vi "GetErrorStructureSize.vi"(8 "error in (no error)":errorcluster) -> (0 "error out":errorcluster, 3 "CS size if BD is empty":T1={"Width (%)"=70.0, "Height (%)"=50.0})   [LabVIEW 2017, in "ErrorStructureDrawer.lvlib"]
doc: "Gets the size at which the new case structure should be drawn if there is nothing to put inside that case structure from the config FGV. Size is specified as a percentage of the size of the visible block diagram."
uses:
  ErrorStructureDrawer.lvlib
  Controls/CaseStructureSizeIfBD_Empty.ctl
  Controls/GetSetCommand.ctl
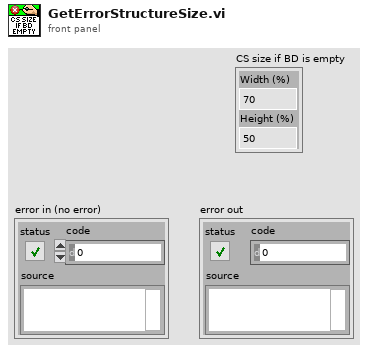
[diagram p1: front panel]
types:
  T1 = typedef "ErrorStructureDrawer.lvlib/CaseStructureSizeIfBD_Empty.ctl" = cluster{"Width (%)":dbl, "Height (%)":dbl}
  T2 = typedef "ErrorStructureDrawer.lvlib/GetSetCommand.ctl" = enum16{"Get", "Set"}
  T3 = typedef "ErrorStructureDrawer.lvlib/ErrorStructureDrawerSettings.ctl" = cluster{"Error control config":T4, "BD alignment settings":T5, "Case structure outer whitespace (px)":T6, "Case structure inner whitespace (px)":T7, "Case structure constants":T8, "CS size if BD is empty":T1}
  T4 = typedef "ErrorStructureDrawer.lvlib/ErrorControlConfig.ctl" = cluster{"Error control path":path, "Error indicator path":path, "Error control vertical spacing from existing FP items":i16, "Error-control to error-indicator horizontal spacing on FP":i16, "Error control vertical spacing from existing BD items":i32, "Error indicator vertical spacing from existing BD items":i32}
  T5 = typedef "ErrorStructureDrawer.lvlib/BD_AlignmentSettings.ctl" = cluster{"Controls":enum32{"Top Edges", "Vertical Centers", "Bottom Edges", "Left Edges", "Horizontal Centers", "Right Edges"}, "Indicators":enum32{"Top Edges", "Vertical Centers", "Bottom Edges", "Left Edges", "Horizontal Centers", "Right Edges"}}
  T6 = typedef "ErrorStructureDrawer.lvlib/CaseStructureOuterWhitespace.ctl" = cluster{"Control terminals right-side":i32, "Indicator terminals left-side":i32}
  T7 = typedef "ErrorStructureDrawer.lvlib/CaseStructureInnerWhitespace.ctl" = cluster{"Left":u32, "Right":u32, "Top":u32, "Bottom":u32}
  T8 = typedef "ErrorStructureDrawer.lvlib/CaseStructureConstants.ctl" = cluster{"Border thickness":u32, "Case-menu height":u32}
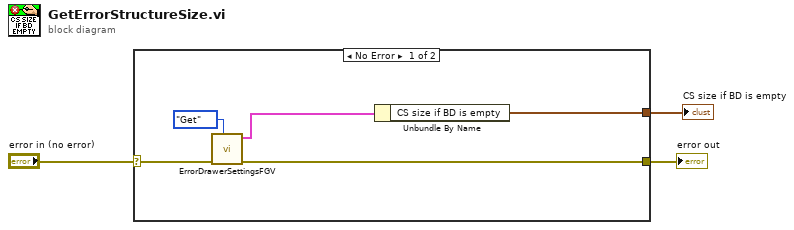
[diagram p0: block diagram]
diagram:
  n1 = case shown="No Error" "error in (no error)" {
    selector: "error in (no error)" -> [w5 w9]
    tunnel: [w8 w9] -> w3
    tunnel: [w4 _] -> w1
    frame No Error {
      n2 = call "ErrorDrawerSettingsFGV.vi"("Get or Set (Get)"=GetSetCommand."Get", "Error In"=w5) -> ("Error Out"=w8:errorcluster, "Error structure drawer settings"=w7:T3)  [unwired: 8 in]
      n3 = Unbundle By Name(w7) -> ("CS size if BD is empty"=w4:T1)
    }
    frame Error {
    }
  }
  "error out" <- w3
  "CS size if BD is empty" <- w1
